vi "initialize photometrics.vi"(8 "error in (no error)":errorcluster, 10 "Temperature":dbl=-25.0, 11 "exposure (s)":dbl=0.04) -> (0 "error out":errorcluster, 2 "error out 2":errorcluster caption="error out", 3 "Camera Handle":u32)   [LabVIEW 2013, in "Ch300Camera.lvclass"]
uses:
  Ch300Camera.lvclass
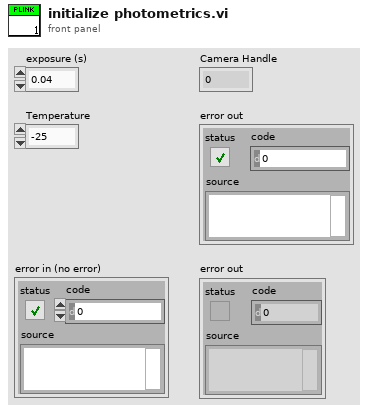
[diagram p1: front panel]
types:
  T1 = cluster{"Time pre open":dbl, "Time poster open":dbl, "Shutter State":u16}
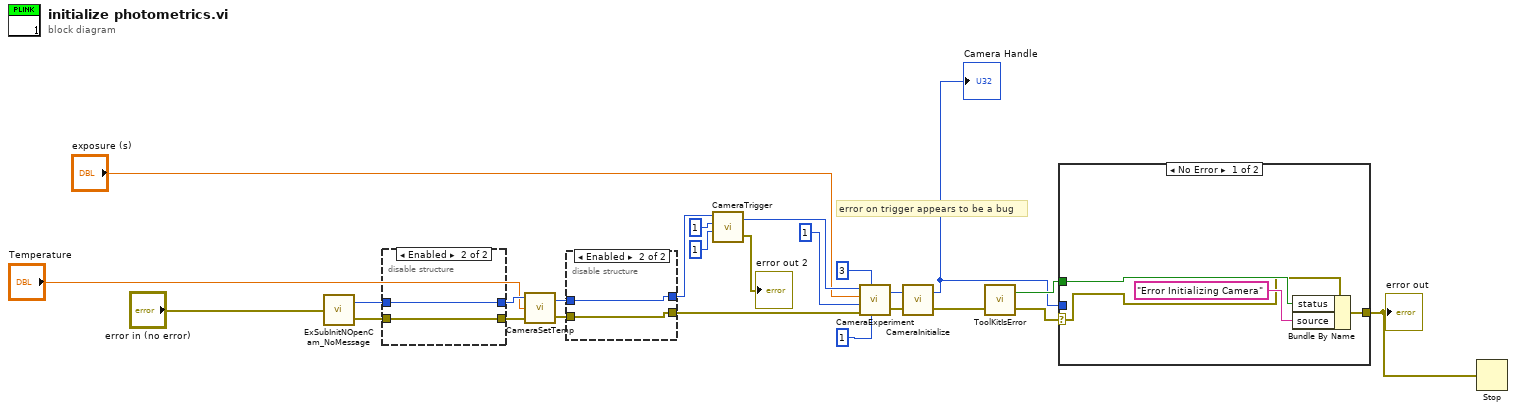
[diagram p0: block diagram]
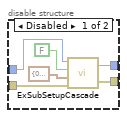
[diagram p2: hidden frame]
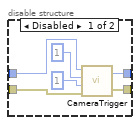
[diagram p3: hidden frame]
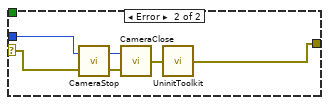
[diagram p4: hidden frame]
diagram:
  # "error on trigger appears to be a bug"
  n1 = call "ExSubInitNOpenCam_NoMessage.vi"("error in (no error)"="error in (no error)") -> ("Camera Handle"=w5:u32, "error out"=w7:errorcluster)
  n2 = disable-structure shown="Enabled" {
    disable-tunnel: w5 -> [w29 w32]
    disable-tunnel: [w28 w32] -> w6
    disable-tunnel: w7 -> [w27 w33]
    disable-tunnel: [w26 w33] -> w8
    frame Disabled {
      n3 = call <userlib>:"CameraTrigger.vi"("error in"=w27, "Trigger Edge"=u32 1, "Timing Mode"=u32 1, "Camera Handle"=w29) -> ("error out"=w26:errorcluster, "Camera Handle"=w28:u32)
    }
    frame Enabled {
    }
  }
  n4 = call <userlib>:"CameraSetTemp.vi"("error in (no error)"=w8, "Temperature"="Temperature", "Camera Handle"=w6) -> ("error out"=w3:errorcluster, "Camera Handle"=w4:u32)
  n5 = disable-structure shown="Enabled" {
    disable-tunnel: w3 -> [w38 w40]
    disable-tunnel: w4 -> [w37 w41]
    disable-tunnel: [w36 w41] -> w14
    disable-tunnel: [w35 w40] -> w24
    frame Disabled {
      n6 = call "ExSubSetupCascade.vi"("error in (no error)"=w38, "Shutter control"=T1 {"Time pre open"=0.0, "Time poster open"=0.0, "Shutter State"=2}, "OverLap Mode"=FALSE, "Camera Handle"=w37) -> ("error out"=w35:errorcluster, "Camera Handle"=w36:u32)
    }
    frame Enabled {
    }
  }
  n7 = call <userlib>:"CameraTrigger.vi"("Trigger Edge"=u32 1, "Timing Mode"=u32 1, "Camera Handle"=w14) -> ("error out"=→"error out 2":errorcluster, "Camera Handle"=w15:u32)  [unwired: 1 in]
  n8 = call <userlib>:"CameraExperiment.vi"("Number of Accumulations"=u32 1, "Acquire / Focus Flag"=u32 3, "error in"=w24, "Number of Images"=u32 1, "Exposure (sec)"="exposure (s)", "Camera Handle"=w15) -> ("error out"=w20:errorcluster, "Camera Handle"=w10:u32)
  n9 = call <userlib>:"CameraInitialize.vi"("error in"=w20, "Camera Handle"=w10) -> ("error out"=w21:errorcluster, "Camera Handle"=w19:u32)
  "Camera Handle" <- w19
  n10 = call <userlib>:"ToolKitIsError.vi"("error in"=w21) -> ("error out"=w1:errorcluster, "Error Flag"=w22:bool)  [unwired: 1 in]
  n11 = case shown="No Error" w1 {
    selector: w1 -> [w42 w47]
    tunnel: [w44 w46] -> w23
    tunnel: w19 -> [_ w48]
    tunnel: w22 -> [w43 _]
    frame No Error {
      n12 = Bundle By Name(cluster=w42, "status"=w43, "source"="Error Initializing Camera") -> (w44:errorcluster)
    }
    frame Error {
      n13 = call <userlib>:"CameraStop.vi"("error in"=w47, "Camera Handle"=w48) -> ("error out"=w49:errorcluster, "Camera Handle"=w50:u32)
      n14 = call <userlib>:"CameraClose.vi"("error in"=w49, "Camera Handle"=w50) -> ("error out"=w51:errorcluster)
      n15 = call <userlib>:"UninitToolkit.vi"("error in"=w51) -> ("error out"=w46:errorcluster)
    }
  }
  "error out" <- w23
  n16 = Stop(stop? (T)=w23) -> ()
